vi "TestHDF5.vi"() -> ()   [LabVIEW 2013]
uses:
  <vilib>/addons/h5labview2/file/H5Fmode.ctl
  <vilib>/addons/h5labview2/base/lib_path.vi
  <vilib>/addons/h5labview2/base/H5Equery.vi
  <vilib>/addons/h5labview2/dataset/H5Dwrite.llb/H5Dwrite.xnode
  <vilib>/addons/h5labview2/file/H5F.lvlib
panel:
  in  "data":dbl[](array[numeric])
  in  "path":path
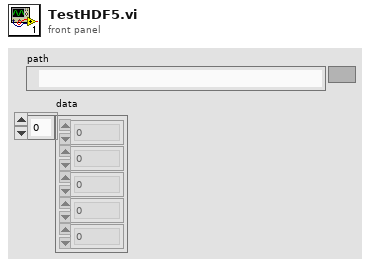
[diagram p1: front panel]
types:
  T1 = typedef "H5F.lvlib/H5Fmode.ctl" = enum16{"read-only", "read-write", "overwrite", "create new", "open or create"}
  T2 = typedef "hid_t.ctl" = i32
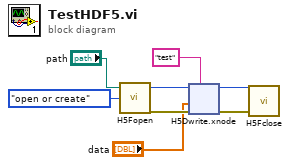
[diagram p0: block diagram]
diagram:
  n1 = call <vilib>:"H5Fopen.vi"("mode (read-only)"=H5Fmode."open or create", "path"="path") -> ("error out"=w4:errorcluster, "ref out"=w6:T2)  [unwired: 2 in]
  n2 = xnode "H5Dwrite.xnode"("dataset name"="test", "error in (no error)"=w4, "data"="data", "ref in"=w6) -> ("error out"=w2:errorcluster, "ref out"=w1:i32)  [unwired: 3 in, 1 out]
  n3 = call <vilib>:"H5Fclose.vi"("error in (no error)"=w2, "ref"=w1) -> ()  [unwired: 3 in, 1 out]
